vi "RichToFlatcif_manager_ErrorInfo.vi"(5 "OutputClusterType":T1, 11 "InputCluster":T2) -> (3 "OutputCluster":T1)   [LabVIEW 2021, in "CIF_Manager_client.lvlib"]
uses:
  cif_manager_ErrorInfo.ctl
  cif_manager_ErrorInfo_Flat.ctl
  CIF_Manager_client.lvlib
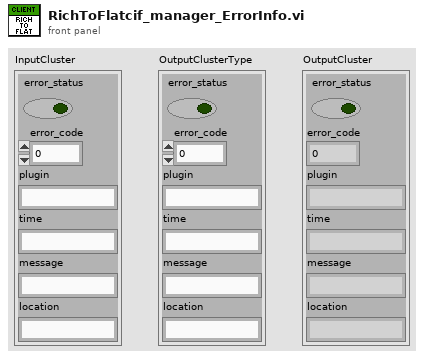
[diagram p1: front panel]
types:
  T1 = typedef "CIF_Manager_client.lvlib/cif_manager_ErrorInfo_Flat.ctl" = cluster{"error_status":bool, "error_code":i32, "plugin":string, "time":string, "message":string, "location":string}
  T2 = typedef "CIF_Manager_client.lvlib/cif_manager_ErrorInfo.ctl" = cluster{"error_status":bool, "error_code":i32, "plugin":string, "time":string, "message":string, "location":string}
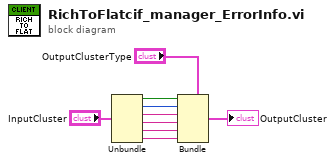
[diagram p0: block diagram]
diagram:
  n1 = Unbundle "Unbundle"("InputCluster") -> ("error_status"=w6:bool, "error_code"=w5:i32, "plugin"=w4:string, "time"=w3:string, "message"=w2:string, "location"=w1:string)
  n2 = Bundle "Bundle"(cluster="OutputClusterType", "error_status"=w6, "error_code"=w5, "plugin"=w4, "time"=w3, "message"=w2, "location"=w1) -> (→"OutputCluster":T1)
